vi "Enable Disable Field Translation.vi"(2 "Disable":bool, 3 "Enable":bool) -> ()   [LabVIEW 2023]
uses:
  <vilib>/Rock Robotics/Network Tables/NT Write Boolean.vi
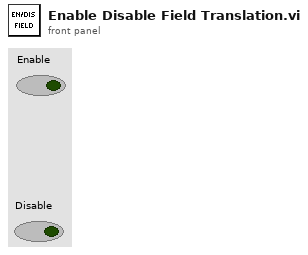
[diagram p1: front panel]
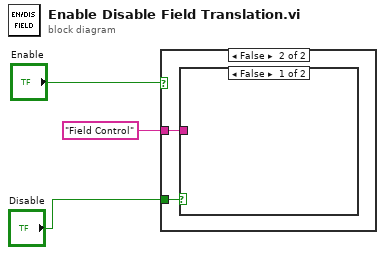
[diagram p0: block diagram]
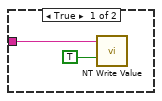
[diagram p2: hidden frame]
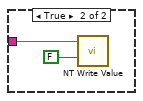
[diagram p3: hidden frame]
diagram:
  n1 = case shown="False" "Enable" {
    tunnel: "Field Control" ("name") -> [w5 w7]
    tunnel: "Disable" -> [_ w6]
    frame True {
      n2 = call-poly <vilib>:"NT Write Value.vi"("value"=TRUE, "name"=w5) -> ()  [unwired: 9 in, 1 out]
    }
    frame False {
      n3 = case shown="False" w6 {
        tunnel: w7 -> [_ w9]
        frame False {
        }
        frame True {
          n4 = call-poly <vilib>:"NT Write Value.vi"("value"=FALSE, "name"=w9) -> ()  [unwired: 9 in, 1 out]
        }
      }
    }
  }
